vi "Query TSP Link Status.vi"(8 "error in (no error)":errorcluster, 11 "VISA resource name":refnum<visa-resource-name>) -> (0 "error out":errorcluster, 2 "TSP Link State":string, 3 "VISA resource name out":refnum<visa-resource-name>)   [LabVIEW 2020, in "Keithley 2600 Series.lvlib"]
doc: "Returns the state of the TSP-Link system state.\n\n<b>Note:</b>\nThis VI is not available on the models 2604B, 2614B, and 2634B."
uses:
  <instrlib>/Keithley 2600 Series/Keithley 2600 Series.lvlib
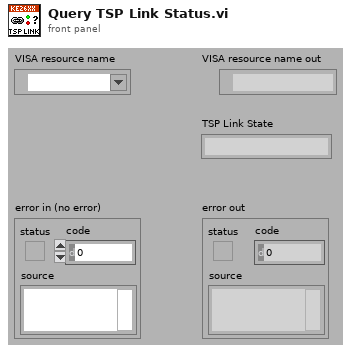
[diagram p1: front panel]
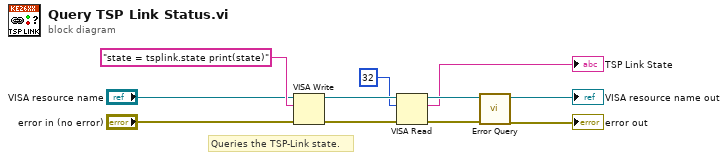
[diagram p0: block diagram]
diagram:
  # "Queries the TSP-Link state."
  n1 = VISA Write(VISA resource name="VISA resource name", write buffer="state = tsplink.state print(state)", error in (no error)="error in (no error)") -> (VISA resource name out=w4:refnum<visa-resource-name>, error out=w3:errorcluster)  [unwired: 1 out]
  n2 = VISA Read(VISA resource name=w4, byte count=u32 32, error in (no error)=w3) -> (VISA resource name out=w5:refnum<visa-resource-name>, read buffer=→"TSP Link State":string, error out=w6:errorcluster)  [unwired: 1 out]
  n3 = call <instrlib>:"Error Query.vi"("error in (no error)"=w6, "VISA resource name"=w5) -> ("error out"=→"error out":errorcluster, "VISA resource name out"=→"VISA resource name out":refnum<visa-resource-name>)  [unwired: 6 in, 2 out]
